vi "Quoter.vi"(1 "String In":string) -> (0 "String Out":string)   [LabVIEW 2014]
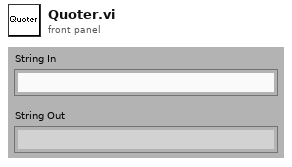
[diagram p1: front panel]
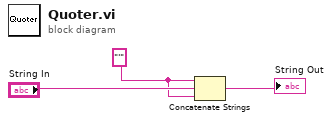
[diagram p0: block diagram]
diagram:
  w1 = "'" ("search string")
  n1 = Concatenate Strings(w1, "String In", w1) -> (→"String Out":string)
